vi "SetParam.vi"(7 "RS":bool, 8 "error in (no error)":errorcluster, 9 "Param to Set in":u16, 10 "Visa":refnum<visa-resource-name>) -> (0 "error out":errorcluster)   [LabVIEW 2017]
uses:
  <vilib>/Utility/miscctls.llb/LVMinMaxIncTypeDef.ctl
panel:
  out "RS Out":string
  out "Horizontal Progress Bar":i32(slide) min=0 max=50 scale=0.0..50.0
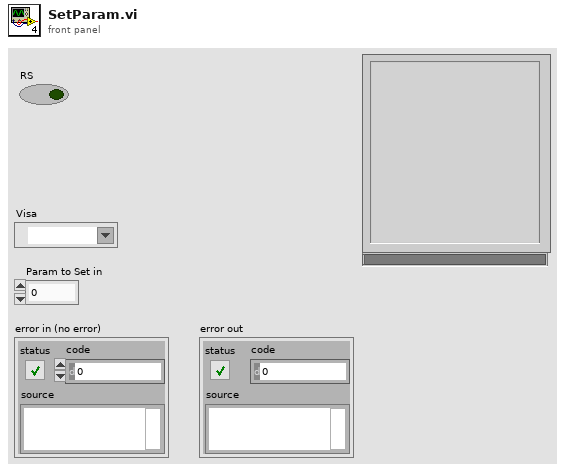
[diagram p1: front panel]
types:
  T1 = typedef "LVMinMaxIncTypeDef.ctl" = cluster{"Minimum":dbl, "Maximum":dbl, "Increment":dbl}
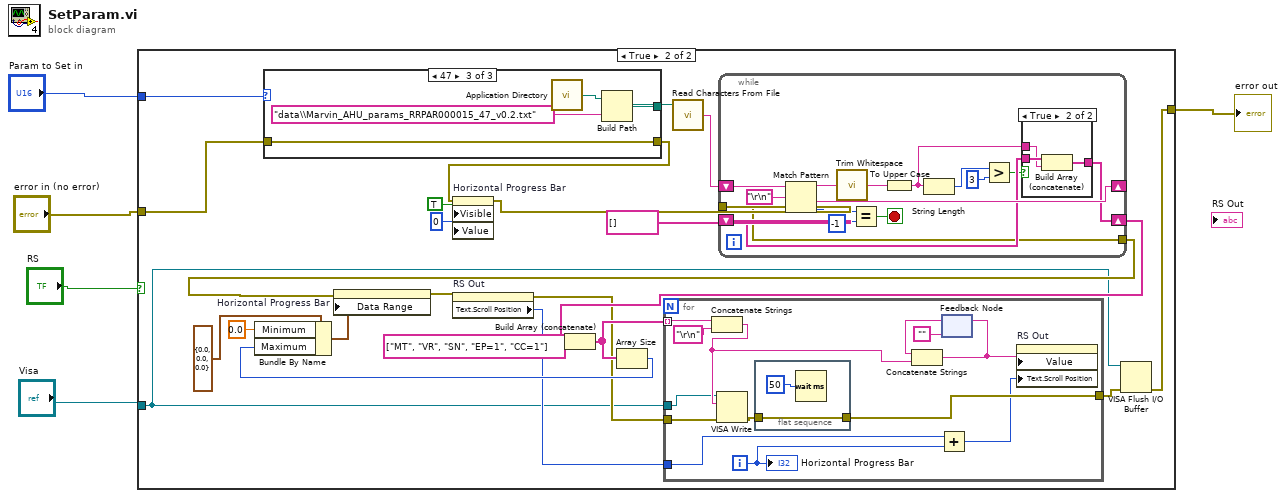
[diagram p0: block diagram]
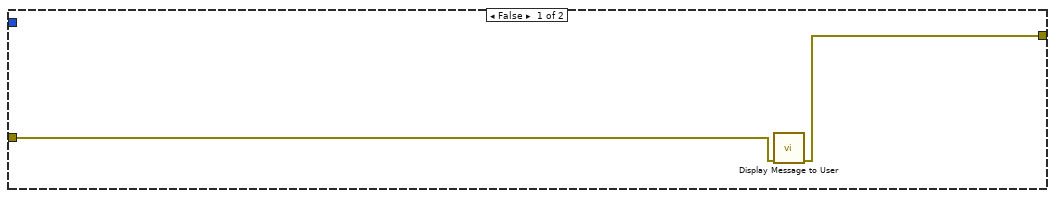
[diagram p2: hidden frame]
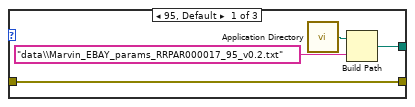
[diagram p4: hidden frame]
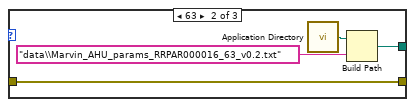
[diagram p5: hidden frame]
diagram:
  n1 = case shown="True" "RS" {
    tunnel: "error in (no error)" -> [w7 w17]
    tunnel: [w6 w14] -> w3
    tunnel: "Visa" -> [_ w9]
    tunnel: "Param to Set in" -> [_ w8]
    frame False {
      n2 = call "Display Message to User"("error in (no error)"=w7) -> ("error out"=w6:errorcluster)  [unwired: 9 in, 1 out]
    }
    frame True {
      n3 = case shown="47" w8 {
        tunnel: [w66 w70 w74] -> w28
        tunnel: w17 -> [w65 w69 w73]
        tunnel: [w65 w69 w73] -> w20
        frame 95, Default {
          n4 = call <vilib>:"Application Directory.vi"() -> ("Application Directory"=w68:path)
          n5 = Build Path(base path=w68, name or relative path="data\\Marvin_EBAY_params_RRPAR000017_95_v0.2.txt") -> (appended path=w66:path)
        }
        frame 63 {
          n6 = call <vilib>:"Application Directory.vi"() -> ("Application Directory"=w72:path)
          n7 = Build Path(base path=w72, name or relative path="data\\Marvin_AHU_params_RRPAR000016_63_v0.2.txt") -> (appended path=w70:path)
        }
        frame 47 {
          n8 = call <vilib>:"Application Directory.vi"() -> ("Application Directory"=w76:path)
          n9 = Build Path(base path=w76, name or relative path="data\\Marvin_AHU_params_RRPAR000015_47_v0.2.txt") -> (appended path=w74:path)
        }
      }
      n10 = property on="Horizontal Progress Bar" class="Slide (strict)"(error in=w20, "Visible"=TRUE, "Value"=u8 0 ("Horizontal Progress Bar")) -> (error out=w16:errorcluster)  [unwired: 1 in, 1 out]
      n11 = call <vilib>:"Read Characters From File.vi"("file path (dialog if empty)"=w28) -> ("character string"=w29:string)  [unwired: 5 in, 3 out]
      n12 = while {
        shift-right: [w57] -> _
        shift-left: w29 -> [w58]
        shift-right: [w53] -> w18
        shift-left: string[] [] -> [w54]
        tunnel: w16 -> [w46]
        tunnel: [w46] -> w10
        stop <- w59 stop-if-true
        n13 = Match Pattern(string=w58, regular expression="\r\n") -> (before substring=w55:string, after substring=w57:string, offset past match=w56:i32)  [unwired: 1 in, 1 out]
        n14 = call <vilib>:"Trim Whitespace.vi"("string"=w55) -> ("trimmed string"=w52:string)  [unwired: 1 in]
        n15 = Equal?(x=w56, y=-1) -> (x = y?=w59:bool)
        n16 = To Upper Case(1:w52) -> (0:w50:string)
        n17 = String Length(string=w50) -> (length=w49:i32)
        n18 = Greater?(x=w49, y=3) -> (0:w47:bool)
        n19 = case shown="True" w47 {
          tunnel: w54 -> [w61 w64]
          tunnel: [w61 w63] -> w53
          tunnel: w50 -> [_ w62]
          frame False {
          }
          frame True {
            n20 = Build Array (concatenate)(w64, w62) -> (w63:string[])
          }
        }
      }
      n21 = Build Array (concatenate)(w18, string[] ["MT", "VR", "SN", "EP=1", "CC=1"] ("array")) -> (w24:string[])
      n22 = Array Size(array=w24) -> (size(s)=w19:i32)
      n23 = Bundle By Name(cluster=T1 {"Minimum"=0.0, "Maximum"=0.0, "Increment"=0.0} ("Data Entry Limits"), "Minimum"=0.0, "Maximum"=w19) -> (w22:T1)
      n24 = property on="Horizontal Progress Bar" class="Slide (strict)"(error in=w10, "Data Range"=w22) -> (error out=w13:errorcluster)  [unwired: 1 in, 1 out]
      n25 = property on="RS Out" class="Str"(error in=w13) -> (error out=w12:errorcluster, "Text.Scroll Position"=w11:u32)  [unwired: 1 in, 1 out]
      n26 = for {
        tunnel: w24 -> [w38] mode=indexing
        tunnel: w12 -> [w43]
        tunnel: [w35] -> w15
        tunnel: w11 -> [w34]
        tunnel: w9 -> [w31]
        i -> [w33]
        n27 = Concatenate Strings(w38, "\r\n" ("string")) -> (w36:string)
        n28 = VISA Write(VISA resource name=w31, write buffer=w36, error in (no error)=w43) -> (error out=w42:errorcluster)  [unwired: 2 out]
        n29 = flat-sequence {
          tunnel: w42 -> [w44]
          tunnel: [w44] -> w35
          frame #0 {
            n30 = Wait (ms)(milliseconds to wait=u32 50) -> ()  [unwired: 1 out]
          }
        }
        n31 = Add(x=w34, y=w33) -> (x+y=w32:u32)
        n32 = feedback #1("") -> (w40:string)
        n33 = Concatenate Strings(w40, w36) -> (w41:string)
        n34 = feedback-in #1(w41) -> ()
        n35 = property on="RS Out" class="Str"("Value"=w41, "Text.Scroll Position"=w32) -> ()  [unwired: 2 in, 2 out]
        "Horizontal Progress Bar" <- w33
      }
      n36 = VISA Flush I/O Buffer(VISA resource name=w9, error in (no error)=w15) -> (error out=w14:errorcluster)  [unwired: 1 in, 1 out]
    }
  }
  "error out" <- w3
